vi "withdraw.vi"(3 "Application ref in":refnum<vi>) -> (1 "Application ref out":refnum<vi>)   [LabVIEW 2021]
uses:
  <userlib>/Nanonis Prog Interface V5/Nanonis Prog Interface.lvlib
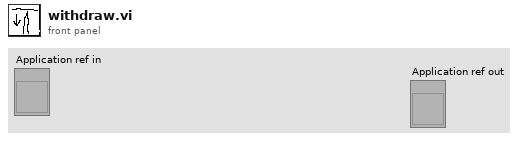
[diagram p1: front panel]
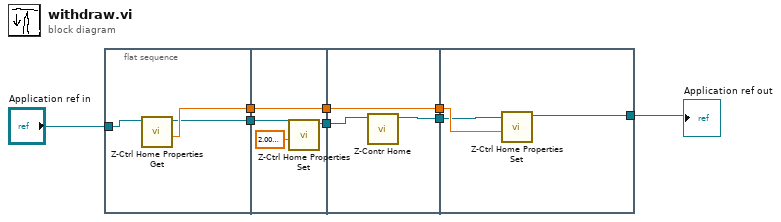
[diagram p0: block diagram]
diagram:
  n1 = flat-sequence {
    tunnel: [w11] -> w6
    tunnel: [w10] -> w5
    tunnel: "Application ref in" -> [w9]
    tunnel: [w14] -> w7
    tunnel: w6 -> [w14]
    tunnel: w5 -> [w13]
    tunnel: [w12] -> w4
    tunnel: [w18] -> w8
    tunnel: w7 -> [w18]
    tunnel: w4 -> [w17]
    tunnel: [w16] -> w3
    tunnel: w8 -> [w21]
    tunnel: w3 -> [w20]
    tunnel: [w19] -> w1
    frame #0 {
      n2 = call <userlib>:"Z-Ctrl Home Properties Get.vi"("Application ref in"=w9) -> ("Home position (m)"=w11:sgl, "Application ref out"=w10:refnum<vi>)  [unwired: 6 in, 2 out]
    }
    frame #1 {
      n3 = call <userlib>:"Z-Ctrl Home Properties Set.vi"("Home position (m) (NaN=no change)"=sgl 2e-07, "Application ref in"=w13) -> ("Application ref out"=w12:refnum<vi>)  [unwired: 7 in, 1 out]
    }
    frame #2 {
      n4 = call <userlib>:"Z-Contr Home.vi"("Application ref in"=w17) -> ("Application ref out"=w16:refnum<vi>)  [unwired: 9 in, 1 out]
    }
    frame #3 {
      n5 = call <userlib>:"Z-Ctrl Home Properties Set.vi"("Home position (m) (NaN=no change)"=w21, "Application ref in"=w20) -> ("Application ref out"=w19:refnum<vi>)  [unwired: 7 in, 1 out]
    }
  }
  "Application ref out" <- w1
